vi "PicoScope5000aExampleAdvancedTriggerV2.vi"() -> ()   [LabVIEW 2010]
doc: "This example demonstrates how to use the PicoScope Labview library to collect data using Advanced triggers in block mode."
uses:
  shared/PicoBuffers.ctl
  <vilib>/Waveform/DWDTOps.llb/DWDT Analog to Digital.vi
  PicoScope5000aLib/PicoScope5000aAnalogChannelSettings.ctl
  shared/Buffer and Transfer Settings.ctl
  shared/Acquisition Settings.ctl
  PicoScope5000aLib/PicoScope5000aDigitalChannelSettings.ctl
panel:
  in  "Pulse Width Qualifier Settings":T1={"Direction"=2, "Lower Limit"=0, "Upper Limit"=0, "Pulse Width Type"=0} {"Pulse Width Type" items=["None", "Less Than", "Greater Than", "In Range", "Out of Range"]; "Direction" items=["Rising"=2, "Falling"=3, "Rising Lower"=7, "Above"=0, "Below"=1, "Rising or Falling"=4, "Falling Lower"=8, "Below Lower"=6, "Above Lower"=5]}
  in  "Trigger Conditions":T2={"Channel A"=1, "Channel B"=0, "Channel C"=0, "Channel D"=0, "Ext"=0, "Aux"=0, "PWQ"=0, "Digital Port 0"=0, "Digital Port 1"=0, "Condition Logic"=0} {"Digital Port 1" items=["Don't Care", "True", "False"]; "Digital Port 0" items=["Don't Care", "True", "False"]; "PWQ" items=["Don't Care", "True", "False"]; "Aux" items=["Don't Care", "True", "False"]; "Ext" items=["Don't Care", "True", "False"]; "Channel D" items=["Don't Care", "True", "False"]; "Channel C" items=["Don't Care", "True", "False"]; "Channel B" items=["Don't Care", "True", "False"]; "Channel A" items=["Don't Care", "True", "False"]; "Condition Logic" items=["AND", "OR", "XOR"]}
  in  "Pulse Width Qualifier Conditions":T3 {"Condition Logic" items=["AND", "OR", "XOR"]}
  in  "Digital Port  0":T4 {"Direction Channel 7" items=["Don't Care", "Low", "High", "Rising", "Falling"]; "Direction Channel 6" items=["Don't Care", "Low", "High", "Rising", "Falling"]; "Direction Channel 5" items=["Don't Care", "Low", "High", "Rising", "Falling"]; "Direction Channel 4" items=["Don't Care", "Low", "High", "Rising", "Falling"]; "Direction Channel 3" items=["Don't Care", "Low", "High", "Rising", "Falling"]; "Direction Channel 2" items=["Don't Care", "Low", "High", "Rising", "Falling"]; "Direction Channel 1" items=["Don't Care", "Low", "High", "Rising", "Falling"]; "Direction Channel 0" items=["Don't Care", "Low", "High", "Rising", "Falling"]}
  in  "Channel A Trigger Properties":T5={"thresholdUpper"=0, "thresholdUpperHysteresis"=0, "thresholdLower"=0, "thresholdLowerHysteresis"=0, "Threshold Mode"=0, "Direction"=2, "Available"=TRUE} {"Direction" items=["Above / Inside", "Below / Outside", "Rising / Enter", "Falling / Exit", "Rising or Falling / Enter or Exit", "Above Lower", "Below Lower", "Rising Lower", "Falling Lower", "Positive Runt", "Negative Runt"]; "Threshold Mode" items=["Level", "Window"]}
  out "overflow":i16 format="%010b"
  in  "Apply Settings":bool
  in  "Port 0 Settings":T6={"Enabled"=FALSE, "Logic Level"=9830} {"Logic Level" items=["1.5V TTL"=9830, "2.5V CMOS"=16383]}
  in  "Channel A Settings":T7={"Enabled"=TRUE, "Coupling"=1, "Range"=6, "Analogue Offset"=0.0, "Bandwidth Limit"=0} {"Bandwidth Limit" items=["Full", "20MHz"]; "Range" items=["10 mV", "20 mV", "50 mV", "100 mV", "200 mV", "500 mV", "1 V", "2 V", "5 V", "10 V", "20 V"]; "Coupling" items=["AC", "DC"]}
  out "USB 3.0 device on non-USB 3.0 Port":bool=TRUE
  out "USB Powered":bool=TRUE
  out "Device Info":T8={"Driver Version"="2.1.104.3324", "USB Version"="2.0", "Hardware"="1", "Variant"="5244A", "Batch and Serial"="CQ178/007", "Cal Date"="11Jun13", "Kernel Version"="1.0", "Digital HW Version"="1", "Analogue HW Version"="1", "MSO"=FALSE, "Number of channels"=2}
  out "error out":errorcluster
  in  "Data file":path=path "PicoScope5000aExampleBlock ChA Data"
  in  "Buffer and Transfer Settings":T9={"startIndex"=0, "Samples"=5000000, "Down Sample Ratio"=1, "Down-Sample Mode"=0} {"Down-Sample Mode" items=["RAW none"=2147483648, "None"=0, "Aggregate"=1, "Decimate"=2, "Average"=4]; "Down Sample Ratio" step=1; "Samples" format="%_6p"}
  in  "Acquisition Settings":T10={"preTriggerSamples"=0, "postTriggerSamples"=5000000, "timebase"=5} {"postTriggerSamples" format="%_6p"; "preTriggerSamples" format="%_6p"}
  out "Properties Panel":T11={"Sample Frequency"=41666668.0, "Sample Rate"=2.4000000209412065e-08, "Max Samples Available"=26843008, "Number of Samples"=0, "Total Capture Time (sec) "=0.0, "Max Total Capture Time Available (sec)"=0.6442322134971619} {"Max Total Capture Time Available (sec)" format="%.3p"; "Sample Frequency" format="%.6p"; "Sample Rate" format="%.3p"; "Max Samples Available" format="%_6p"; "Total Capture Time (sec)" format="%.3p"}
  out "Port 0":digitalwaveform(graph)={"t0"=timestamp(0 s since 1904-01-01), "dt"=8e-09, "Y"={"transitions"=[], "data"=[]}}
  in  "stop":bool
  out "Analog Channels":cluster{i32, sgl, "Data":dbl[]}[](graph)
  in  "Resolution":u32(ring) items=["8-bit"=0, "12-bit"=1, "14-bit"=2, "15-bit"=3, "16-bit"=4, "10-bit"=10]
  in  "Serial Number":string
  in  "Use Serial Number":bool
  in  "error in (no error)":errorcluster
  # "Bit 0 = ChA"
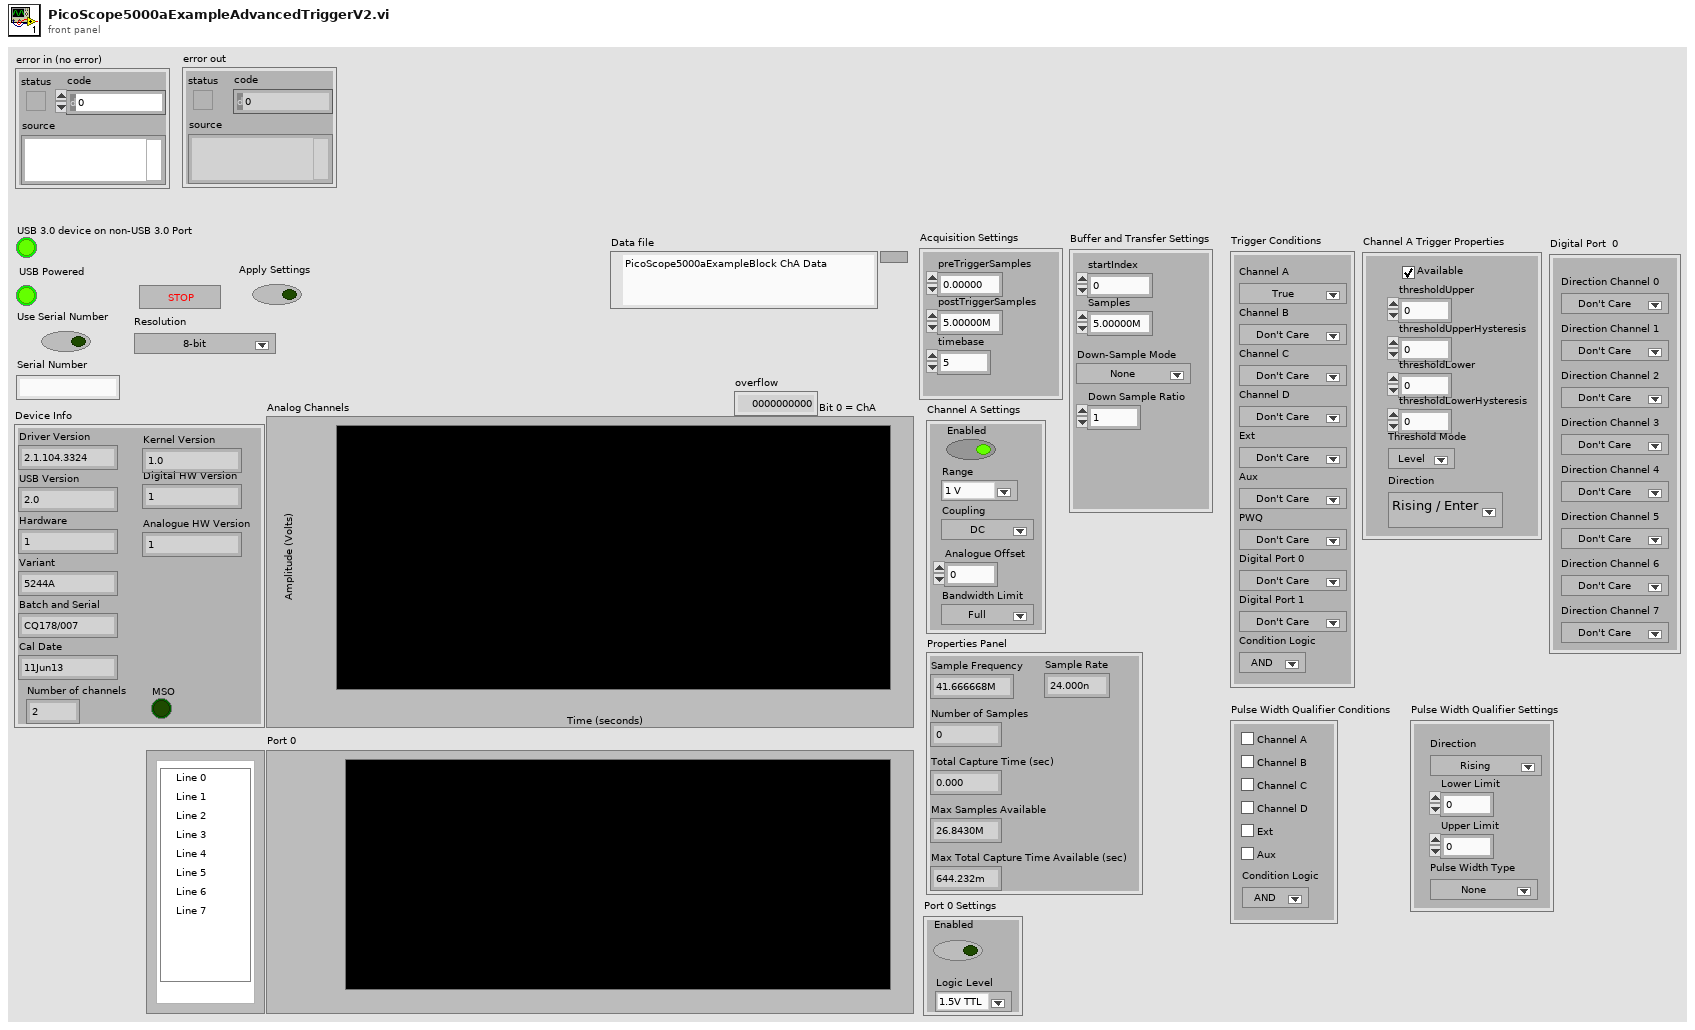
[diagram p1: front panel]
types:
  T1 = cluster{"Direction":u32, "Lower Limit":u32, "Upper Limit":u32, "Pulse Width Type":u32}
  T2 = cluster{"Channel A":u16, "Channel B":u16, "Channel C":u16, "Channel D":u16, "Ext":u16, "Aux":u16, "PWQ":u16, "Digital Port 0":u16, "Digital Port 1":u16, "Condition Logic":u16}
  T3 = cluster{"Channel A":bool, "Channel B":bool, "Channel C":bool, "Channel D":bool, "Aux":bool, "Condition Logic":u16, "Ext":bool}
  T4 = cluster{"Direction Channel 0":u16, "Direction Channel 1":u16, "Direction Channel 2":u16, "Direction Channel 3":u16, "Direction Channel 4":u16, "Direction Channel 5":u16, "Direction Channel 6":u16, "Direction Channel 7":u16}
  T5 = cluster{"thresholdUpper":i16, "thresholdUpperHysteresis":u16, "thresholdLower":i16, "thresholdLowerHysteresis":u16, "Threshold Mode":i32, "Direction":i32, "Available":bool}
  T6 = typedef "PicoScope5000aDigitalChannelSettings.ctl" = cluster{"Enabled":bool, "Logic Level":i16}
  T7 = typedef "PicoScope5000aAnalogChannelSettings.ctl" = cluster{"Enabled":bool, "Coupling":i16, "Range":u16, "Analogue Offset":sgl, "Bandwidth Limit":u32}
  T8 = cluster{"Driver Version":string, "USB Version":string, "Hardware":string, "Variant":string, "Batch and Serial":string, "Cal Date":string, "Kernel Version":string, "Digital HW Version":string, "Analogue HW Version":string, "MSO":bool, "Number of channels":i16}
  T9 = typedef "Buffer and Transfer Settings.ctl" = cluster{"startIndex":u64, "Samples":u64, "Down Sample Ratio":u64, "Down-Sample Mode":u32}
  T10 = typedef "Acquisition Settings.ctl" = cluster{"preTriggerSamples":u64, "postTriggerSamples":u64, "timebase":u32}
  T11 = cluster{"Sample Frequency":dbl, "Sample Rate":dbl, "Max Samples Available":u64, "Number of Samples":u64, "Total Capture Time (sec) ":dbl, "Max Total Capture Time Available (sec)":dbl}
  T12 = enum16{"open", "open or create", "create or replace", "create", "open (read-only)"}
  T13 = typedef "PicoBuffers.ctl" = cluster{"Max Buffer Pointers":u64[][][], "Min Buffer Pointers":u64[][][], "StreamingDataInfo":cluster{"Channel":u32, "Down-Sample Mode":u32, "PICO_DATA_TYPE":enum32{"PICO_INT8_T", "PICO_INT16_T", "PICO_INT32_T", "PICO_UINT32_T", "PICO_INT64_T", ""}, "Samples":i32, "bufferIndex":u64, "startIndex":i32, "overflow":i16}[][]}
  T14 = cluster{"Sample Frequency":sgl, "Sample Rate":sgl, "Max Samples Available":i32, "Number of Samples":u32, "Total Capture Time (sec) ":sgl, "Max Total Capture Time Available (sec)":sgl}
  T15 = cluster{"Channel A Buffer":i16[], "Channel B Buffer":i16[], "Channel C Buffer":i16[], "Channel D Buffer":i16[], "Channel E Buffer":i16[], "Channel F Buffer":i16[], "Channel G Buffer":i16[], "Channel H Buffer":i16[], "Port 0 Buffer":i16[], "Port 1 Buffer":i16[]}[]
  T16 = cluster{"Channel A Buffer":i16[], "Channel B Buffer":i16[], "Channel C Buffer":i16[], "Channel D Buffer":i16[], "Channel E Buffer":i16[], "Channel F Buffer":i16[], "Channel G Buffer":i16[], "Channel H Buffer":i16[], "Port 0 Buffer":i16[], "Port 1 Buffer":i16[]}
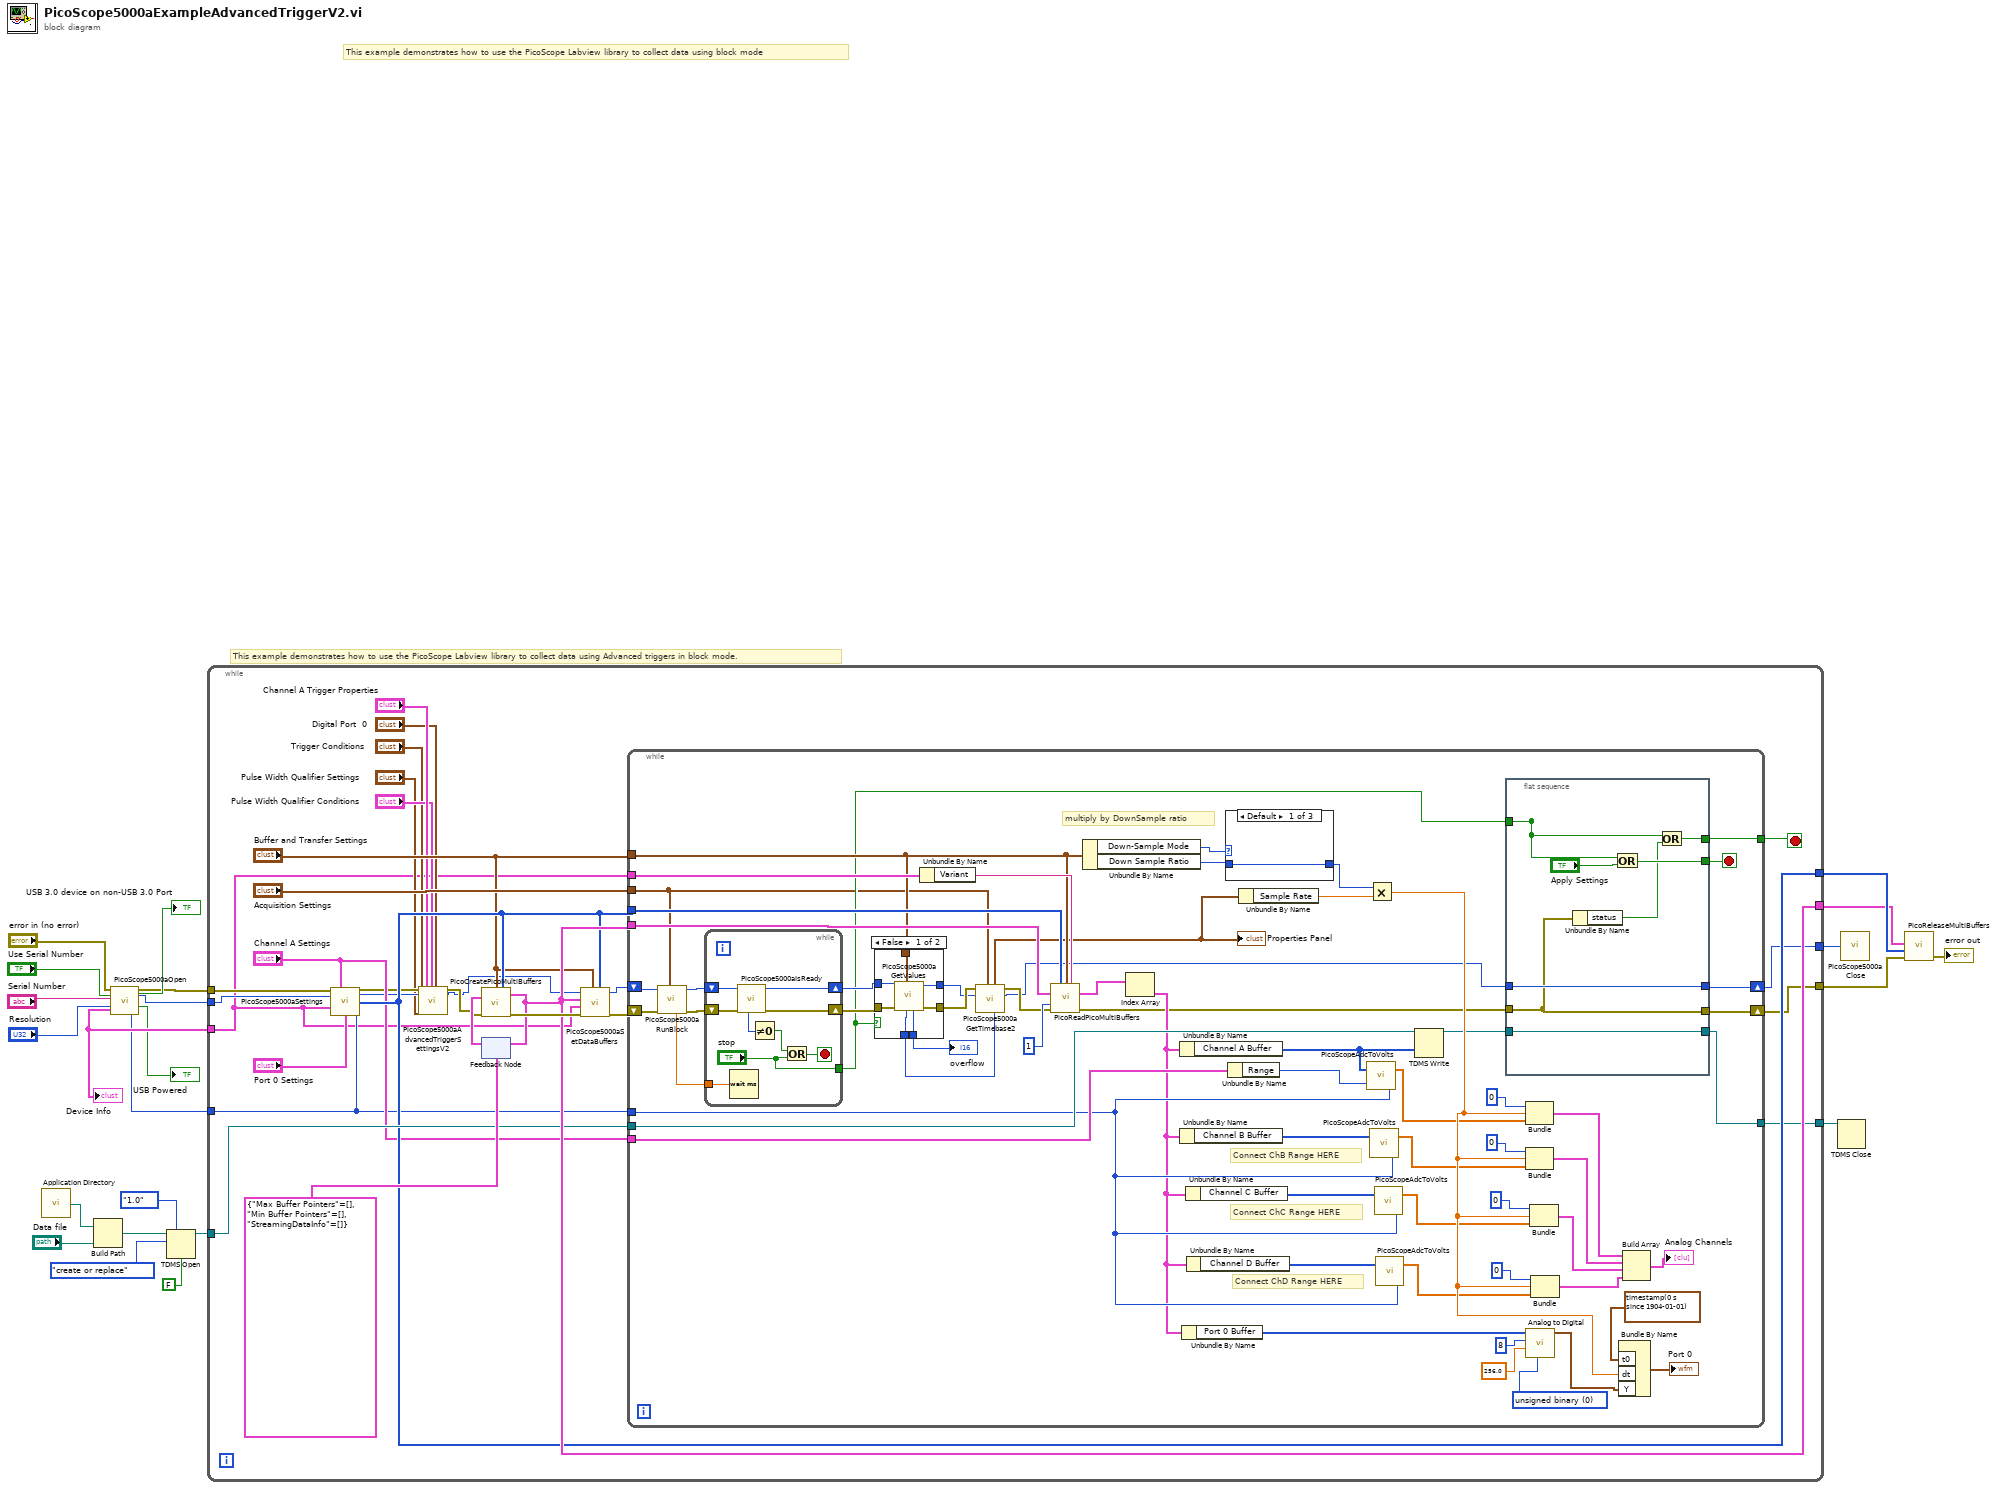
[diagram p0: block diagram]
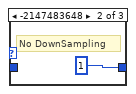
[diagram p3: hidden frame]
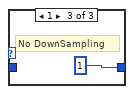
[diagram p4: hidden frame]
diagram:
  # "This example demonstrates how to use the PicoScope Labview library to collect data using Advanced triggers in block mode."
  # "This example demonstrates how to use the PicoScope Labview library to collect data using block mode"
  n1 = call <vilib>:"Application Directory.vi"() -> ("Application Directory"=w15:path)
  n2 = Build Path(base path=w15, name or relative path="Data file") -> (appended path=w16:path)
  n3 = call "PicoScope5000aOpen.vi"("error in (no error)"="error in (no error)", "Serial Number"="Serial Number", "Use Serial Number"="Use Serial Number", "Resolution"="Resolution") -> ("USB 3.0 device on non-USB 3.0 Port"=→"USB 3.0 device on non-USB 3.0 Port":bool, "error out"=w3:errorcluster, "handle"=w23:i16, "USB Powered"=→"USB Powered":bool, "Device Info"=w7:T8, "Max ADC value"=w6:i16)  [unwired: 6 in]
  "Device Info" <- w7
  n4 = TDMS Open(6:FALSE ("disable buffering? (T)"), 7:enum16{"1.0", "2.0"}."1.0" ("file format version (2.0)"), 10:T12."create or replace" ("operation (0:open)"), 11:w16) -> (3:w13:refnum<k34>)  [unwired: 2 in, 1 out]
  n5 = while {
    tunnel: w23 -> [w47]
    tunnel: w6 -> [w41]
    tunnel: [w45] -> w22
    tunnel: [w49] -> w21
    tunnel: [w39] -> w14
    tunnel: w13 -> [w48]
    tunnel: w7 -> [w24]
    tunnel: w3 -> [w46]
    tunnel: [w40] -> w2
    tunnel: [w37] -> w1
    stop <- w38 stop-if-true
    n6 = call "PicoScope5000aSettings.vi"("error in"=w46, "Channel A Settings"="Channel A Settings", "Port 0 Settings"="Port 0 Settings", "handle in"=w47, "Device Info"=w24, "Max ADC value"=w41) -> ("error out"=w33:errorcluster, "handle out"=w30:i16, "enabled array"=w45:i16[])  [unwired: 7 in]
    n7 = call "PicoScope5000aAdvancedTriggerSettingsV2.vi"("error in"=w33, "handle in"=w30, "Trigger Conditions"="Trigger Conditions", "Channel A Trigger Properties"="Channel A Trigger Properties", "Digital Port  0"="Digital Port  0", "Pulse Width Qualifier Conditions"="Pulse Width Qualifier Conditions", "Pulse Width Qualifier Settings"="Pulse Width Qualifier Settings") -> ("error out"=w32:errorcluster, "handle out"=w31:i16)  [unwired: 11 in]
    n8 = feedback #1(T13 {"Max Buffer Pointers"=[], "Min Buffer Pointers"=[], "StreamingDataInfo"=[]} ("Data Pointers")) -> (w51:T13)
    n9 = call "PicoCreatePicoMultiBuffers.vi"("Buffer and Transfer Settings"="Buffer and Transfer Settings", "enabled array"=w45, "Data Pointers In"=w51, "error in (no error)"=w32) -> ("Data Pointers"=w49:T13, "error out"=w50:errorcluster)  [unwired: 10 in]
    n10 = feedback-in #1(w49) -> ()
    n11 = call "PicoScope5000aSetDataBuffers.vi"("enabled array"=w45, "Buffer and Transfer Settings"="Buffer and Transfer Settings", "error in (no error)"=w50, "Device Info"=w24, "Data Pointers In"=w49, "handle in"=w31) -> ("error out"=w36:errorcluster, "handle out"=w35:i16)  [unwired: 4 in]
    n12 = while {
      tunnel: w49 -> [w116]
      tunnel: "Buffer and Transfer Settings" -> [w62]
      tunnel: w45 -> [w107]
      tunnel: "Channel A Settings" -> [w106]
      tunnel: "Acquisition Settings" -> [w53]
      tunnel: w41 -> [w105]
      tunnel: w24 -> [w102]
      tunnel: [w69] -> w38
      shift-right: [w73] -> w40
      shift-left: w36 -> [w63]
      shift-right: [w67] -> w37
      shift-left: w35 -> [w64]
      tunnel: w48 -> [w115]
      tunnel: [w71] -> w39
      stop <- w68 stop-if-true
      w90 = u16 0 items=["unsigned binary", "offset binary", "2's complement"] ("data format (offset binary)")
      # "Connect ChB Range HERE"
      # "Connect ChD Range HERE"
      # "Connect ChC Range HERE"
      # "multiply by DownSample ratio"
      n13 = call "PicoScope5000aRunBlock.vi"("Acquisition Settings"=w53, "error in (no error)"=w63, "handle in"=w64) -> ("error out"=w109:errorcluster, "handle out"=w108:i16, "timeIndisposedMs"=w100:dbl)  [unwired: 5 in, 1 out]
      n14 = while {
        shift-right: [w141] -> w65
        shift-left: w109 -> [w142]
        shift-right: [w140] -> w66
        shift-left: w108 -> [w139]
        tunnel: ["stop"] -> w61
        tunnel: w100 -> [w134]
        stop <- w136 stop-if-true
        n15 = Wait (ms)(milliseconds to wait=w134) -> ()  [unwired: 1 out]
        n16 = call "PicoScope5000aIsReady.vi"("error in (no error)"=w142, "handle in"=w139) -> ("error out"=w141:errorcluster, "handle out"=w140:i16, "ready"=w138:i16)  [unwired: 7 in]
        n17 = Not Equal To 0?(x=w138) -> (x != 0?=w137:bool)
        n18 = Or(x=w137, y="stop") -> (x .or. y?=w136:bool)
      }
      n19 = case shown="False" w61 {
        tunnel: w65 -> [w123 w124]
        tunnel: w66 -> [w122 w125]
        tunnel: [w121 w125] -> w58
        tunnel: [w120 w124] -> w59
        tunnel: w62 -> [w119 _]
        tunnel: [w118 _] -> w60
        tunnel: [w117 _] -> w55
        frame False {
          n20 = call "PicoScope5000aGetValues.vi"("Buffer and Transfer Settings"=w119, "error in (no error)"=w123, "handle in"=w122) -> ("error out"=w120:errorcluster, "handle out"=w121:i16, "overflow"=w118:i16, "noOfSamples"=w117:u64)  [unwired: 5 in]
        }
        frame True {
        }
      }
      "overflow" <- w60
      n21 = Unbundle By Name(w102) -> ("Variant"=w103:string)
      n22 = call "PicoScope5000aGetTimebase2.vi"("Number of Samples"=w55, "Acquisition Settings"=w53, "handle in"=w58, "error in (no error)"=w59) -> ("handle out"=w56:i16, "error out"=w57:errorcluster, "Properties Panel"=w54:T14)  [unwired: 5 in]
      "Properties Panel" <- w54
      n23 = call "PicoReadPicoMultiBuffers.vi"("enabled array"=w107, "Buffer and Transfer Settings"=w62, "Variant"=w103, "Data Pointers"=w116, "No of Buffers"=1, "error in (no error)"=w57) -> ("MultiBuffers (Max or non-aggregated)"=w114:T15, "error out"=w70:errorcluster)  [unwired: 7 in, 1 out]
      n24 = Unbundle By Name(w62) -> ("Down-Sample Mode"=w112:u32, "Down Sample Ratio"=w113:u64)
      n25 = Index Array(array=w114) -> (element=w74:T16)  [unwired: 1 in]
      n26 = Unbundle By Name(w74) -> ("Channel A Buffer"=w83:i16[])
      n27 = Unbundle By Name(w74) -> ("Channel B Buffer"=w96:i16[])
      n28 = Unbundle By Name(w74) -> ("Port 0 Buffer"=w88:i16[])
      n29 = Unbundle By Name(w74) -> ("Channel C Buffer"=w81:i16[])
      n30 = Unbundle By Name(w74) -> ("Channel D Buffer"=w77:i16[])
      n31 = case shown="Default" w112 {
        tunnel: [w143 u64 1 ("Down Sample Ratio") u64 1 ("Down Sample Ratio")] -> w110
        tunnel: w113 -> [w143 _ _]
        frame Default {
        }
        frame -2147483648 {
          # "No DownSampling"
        }
        frame 1 {
          # "No DownSampling"
        }
      }
      n32 = Unbundle By Name(w106) -> ("Range"=w98:u16)
      n33 = Unbundle By Name(w54) -> ("Sample Rate"=w104:sgl)
      n34 = call "PicoScopeAdcToVolts.vi"("Max_adc"=w105, "Range Index"=w98, "Data"=w83) -> ("Data"=w84:dbl[])
      n35 = Multiply(x=w110, y=w104) -> (x*y=w111:sgl)
      n36 = call "PicoScopeAdcToVolts.vi"("Max_adc"=w105, "Data"=w96) -> ("Data"=w95:dbl[])  [unwired: 1 in]
      n37 = call "PicoScopeAdcToVolts.vi"("Max_adc"=w105, "Data"=w81) -> ("Data"=w80:dbl[])  [unwired: 1 in]
      n38 = call "PicoScopeAdcToVolts.vi"("Max_adc"=w105, "Data"=w77) -> ("Data"=w76:dbl[])  [unwired: 1 in]
      n39 = TDMS Write(0:w115, 9:w83) -> (4:w72:refnum<k34>)  [unwired: 4 in, 3 out]
      n40 = flat-sequence {
        tunnel: [w133] -> w68
        tunnel: [w126] -> _
        tunnel: [w130] -> w69
        tunnel: w56 -> [w129]
        tunnel: [w129] -> w67
        tunnel: w70 -> [w128]
        tunnel: [w128] -> w73
        tunnel: [w127] -> w71
        tunnel: w72 -> [w127]
        tunnel: w61 -> [w126]
        frame #0 {
          n41 = Unbundle By Name(w128) -> ("status"=w131:bool)
          n42 = Or(x=w126, y="Apply Settings") -> (x .or. y?=w133:bool)
          n43 = Or(x=w126, y=w131) -> (x .or. y?=w130:bool)
        }
      }
      n44 = Bundle(0, w111, "Data"=w84) -> (w94:cluster{i32, sgl, "Data":dbl[]})  [unwired: 1 in]
      n45 = Bundle(0, w111, "Data"=w95) -> (w93:cluster{i32, sgl, "Data":dbl[]})  [unwired: 1 in]
      n46 = call-poly <vilib>:"Analog to Digital.vi"("data format (offset binary)"=w90, "full-scale range (pk-pk)"=256.0, "resolution (16 bit)"=8, "analog waveform"=w88) -> ("digital waveform"=w85:digitalwaveform)  [unwired: 4 in, 3 out]
      n47 = Bundle(0, w111, "Data"=w80) -> (w79:cluster{i32, sgl, "Data":dbl[]})  [unwired: 1 in]
      n48 = Bundle(0, w111, "Data"=w76) -> (w75:cluster{i32, sgl, "Data":dbl[]})  [unwired: 1 in]
      n49 = Bundle By Name("t0"=timestamp(0 s since 1904-01-01), "dt"=w111, "Y"=w85) -> (→"Port 0":digitalwaveform)  [unwired: 1 in]
      n50 = Build Array(w94, w93, w79, w75) -> (→"Analog Channels":cluster{i32, sgl, "Data":dbl[]}[])
    }
  }
  n51 = TDMS Close(11:w14) -> ()  [unwired: 1 in, 2 out]
  n52 = call "PicoScope5000aClose.vi"("handle"=w1) -> ()
  n53 = call "PicoReleaseMultiBuffers.vi"("error in (no error)"=w2, "Enabled array"=w22, "Data Pointers"=w21) -> ("error out"=→"error out":errorcluster)  [unwired: 7 in, 1 out]
